vi "PostInit.vi"(8 "error in (no error)":errorcluster, 11 "Bouncer in":refnum<class "Bouncer.lvclass">) -> (0 "error out":errorcluster, 3 "Bouncer out":refnum<class "Bouncer.lvclass">)   [LabVIEW 2019, in "RT_Game.lvlib" / "Bouncer.lvclass"]
uses:
  Bouncer.lvclass
  C:/Users/FreshBob/Dropbox/VIs/myRIO_GameConsole/RT/RT_Game/Game/Game.lvclass
  Game/SpritesCluster.ctl
  RT_Sprite/RT_Sprite.lvclass
  Bouncer.lvclass/Bouncer.ctl
  PongPanel/PongPanel.lvclass
  C:/Users/FreshBob/Dropbox/VIs/myRIO_GameConsole/RT/RT_Game/RT_Sprite/RT_Sprite.lvclass
  PongBall/PongBall.lvclass
  Game/Game.lvclass
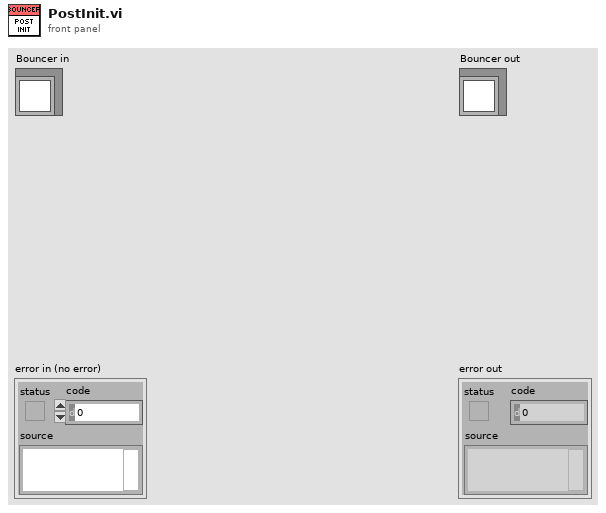
[diagram p1: front panel]
types:
  T1 = typedef "RT_Game.lvlib/Game.lvclass/SpritesCluster.ctl" = cluster{"Sprite1":refnum<class "RT_Sprite.lvclass">, "Sprite2":refnum<class "RT_Sprite.lvclass">, "Sprite3":refnum<class "RT_Sprite.lvclass">}
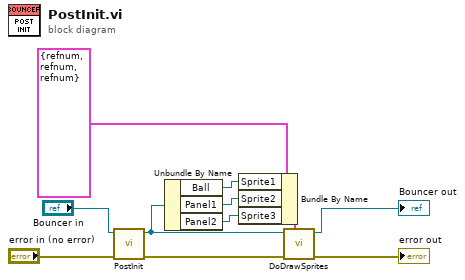
[diagram p0: block diagram]
diagram:
  n1 = call-parent "PostInit.vi"("error in (no error)"="error in (no error)", "Game in"="Bouncer in") -> ("error out"=w11:errorcluster, "Game out"=w2:refnum<class "Bouncer.lvclass">)  [unwired: 8 in]
  n2 = Unbundle By Name(w2) -> ("Ball"=w4:refnum<class "PongBall.lvclass">, "Panel1"=w3:refnum<class "PongPanel.lvclass">, "Panel2"=w1:refnum<class "PongPanel.lvclass">)
  n3 = Bundle By Name(cluster=T1 {"Sprite1"=refnum, "Sprite2"=refnum, "Sprite3"=refnum} ("Sprites in"), "Sprite1"=w4, "Sprite2"=w3, "Sprite3"=w1) -> (w5:T1)
  n4 = call "DoDrawSprites.vi"("error in (no error)"=w11, "Sprites in"=w5, "Game in"=w2) -> ("error out"=→"error out":errorcluster, "Game out"=→"Bouncer out":refnum<class "Bouncer.lvclass">)  [unwired: 6 in, 1 out]
